vi "Sort active pickup area.vi"(2 "Insect-data-array":dbl[][](array[numeric])) -> (0 "Insect-data-array (out of range removed)":dbl[][](array[numeric]))   [LabVIEW 2024]
doc: "Removes insects from array that are outside ithe pickup area"
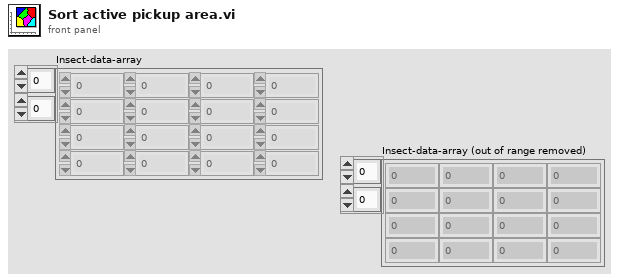
[diagram p1: front panel]
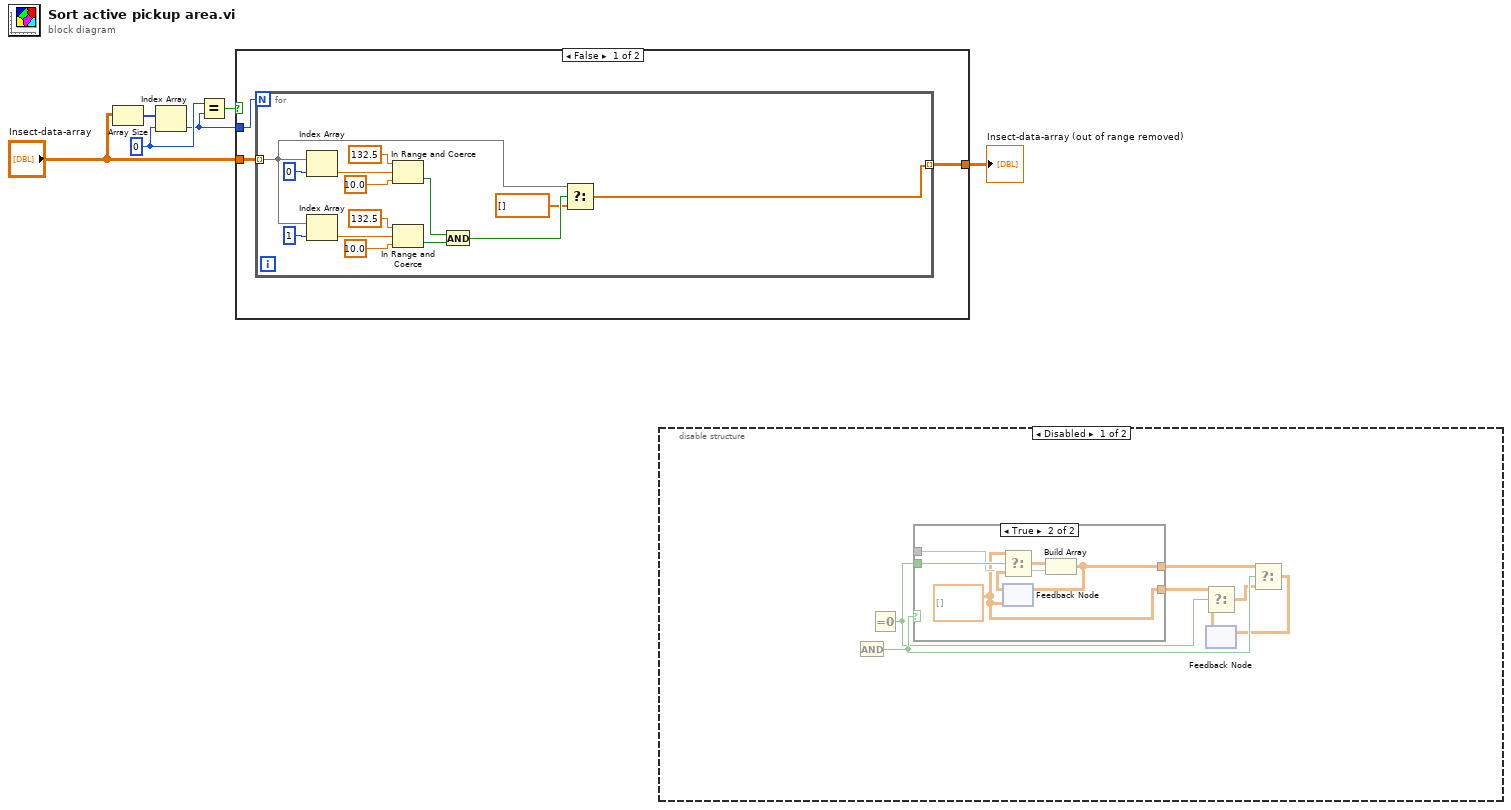
[diagram p0: block diagram]
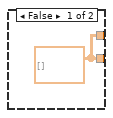
[diagram p2: hidden frame]
diagram:
  w3 = 0 ("index")
  n1 = Array Size(array="Insect-data-array") -> (size(s)=w6:i32[])
  n2 = Index Array(array=w6, index=w3) -> (element=w2:i32)
  n3 = Equal?(x=w3, y=w2) -> (x = y?=w1:bool)
  n4 = case shown="False" w1 {
    tunnel: "Insect-data-array" -> [w9 w24]
    tunnel: w2 -> [w8 _]
    tunnel: [w7 w24] -> w4
    frame False {
      n5 = for {
        N: w8 -> [_]
        tunnel: w9 -> [w13] mode=indexing
        tunnel: [w10] -> w7 mode=indexing
        n6 = Index Array(array=w13, index=0) -> (element=w17:dbl)
        n7 = Index Array(array=w13, index=1) -> (element=w16:dbl)
        n8 = In Range and Coerce(upper limit=132.5, x=w17, lower limit=10.0) -> (In Range?=w15:bool)  [unwired: 1 out]
        n9 = In Range and Coerce(upper limit=132.5, x=w16, lower limit=10.0) -> (In Range?=w14:bool)  [unwired: 1 out]
        n10 = And(x=w15, y=w14) -> (x .and. y?=w12:bool)
        n11 = Select(t=w13, s=w12, f=dbl[] []) -> (s? t:f=w10:dbl[])
      }
    }
    frame True {
    }
  }
  "Insect-data-array (out of range removed)" <- w4
  n12 = disable-structure shown="Disabled" {
    frame Disabled {
      n13 = And() -> (x .and. y?=w31:bool)  [unwired: 2 in]
      n14 = Equal To 0?() -> (x = 0?=w28:bool)  [unwired: 1 in]
      n15 = case shown="True" w31 {
        tunnel: w28 -> [_ w38]
        tunnel: _ -> [_ w35]
        tunnel: [w32 w34] -> w30
        tunnel: [w32 w33] -> w27
        frame False {
          w32 = dbl[][] []
        }
        frame True {
          w33 = dbl[][] []
          n16 = feedback #1(w33) -> (w36:dbl[][])
          n17 = Select(t=w33, s=w38, f=w36) -> (s? t:f=w37:dbl[][])
          n18 = Build Array(w37, w35) -> (w34:dbl[][][])
          n19 = feedback-in #1(w34) -> ()
        }
      }
      n20 = feedback #2() -> (w26:dbl[][][])  [unwired: 1 in]
      n21 = Select(t=w27, s=w28, f=w26) -> (s? t:f=w25:dbl[][])
      n22 = Select(t=w30, s=w31, f=w25) -> (s? t:f=w29:dbl[][][])
      n23 = feedback-in #2(w29) -> ()
    }
    frame Enabled {
    }
  }
